vi "Read Characteristics array.vi"(8 "error in (no error)":errorcluster, 11 "Analysis params in":refnum<class "CV-Analysis.lvclass">) -> (0 "error out":errorcluster, 2 "Characteristics array":T1[](array[typedef]), 3 "Analysis params out":refnum<class "CV-Analysis.lvclass">)   [LabVIEW 2013, in "CameraVision.lvlib" / "CV-Analysis.lvclass"]
uses:
  CV-Analysis.lvclass
  Characteristics-cluster.ctl
  CV-Analysis.lvclass/CV-Analysis.ctl
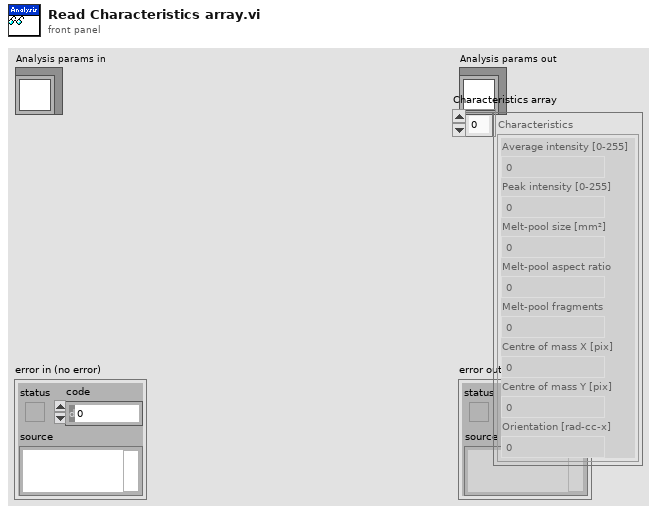
[diagram p1: front panel]
types:
  T1 = typedef "CameraVision.lvlib/CV-Analysis.lvclass/Characteristics-cluster.ctl" = cluster{"Average intensity":dbl, "Peak intensity":dbl, "Melt-pool size":dbl, "Melt-pool aspect ratio":dbl, "Melt-pool fragments":dbl, "Centre of mass X":dbl, "Centre of mass Y":dbl, "Orientation":dbl}
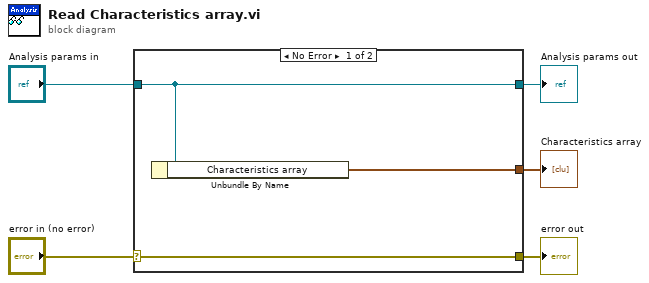
[diagram p0: block diagram]
diagram:
  n1 = case shown="No Error" "error in (no error)" {
    selector: "error in (no error)" -> [w8 w9]
    tunnel: [w8 w9] -> w4
    tunnel: [w7 w10] -> w2
    tunnel: "Analysis params in" -> [w7 w10]
    tunnel: [w6 _] -> w1
    frame No Error {
      n2 = Unbundle By Name(w7) -> ("Characteristics array"=w6:T1[])
    }
    frame Error {
    }
  }
  "error out" <- w4
  "Analysis params out" <- w2
  "Characteristics array" <- w1
